vi "ep_Rapid Voltage Changes (1ch).vi"(0 "RMS (1/2) (half cycle)":cluster{"times":timestamp[], "RMS (1/2)":dbl[]}, 1 "init":bool, 5 "RVC settings":T3={"min rate of change [%/sec]"=0.5, "steadiness of steady state [%]"=0.2, "min steady state duration [sec]"=1.0, "min steady state difference [%]"=0.0, "max voltage change [%]"=3.3}, 7 "voltage flag":bool, 9 "nominal voltage [V]":dbl=230.0, 11 "phase":T1, 12 "nominal frequency":enum16{"50 Hz", "60 Hz"}(ring)) -> (4 "rapid voltage changes":T2(array[cluster]), 6 "d(t)":dbl[](array[numeric]))   [LabVIEW 2011, in "NI_EP_Power Quality.lvlib"]
uses:
  <vilib>/addons/Electrical Power/PQ/NI_EP_Power Quality.lvlib
  <vilib>/addons/Electrical Power/PQ/Common/Controls/ep_Phase.ctl
  <vilib>/Analysis/NI_AALBase.lvlib
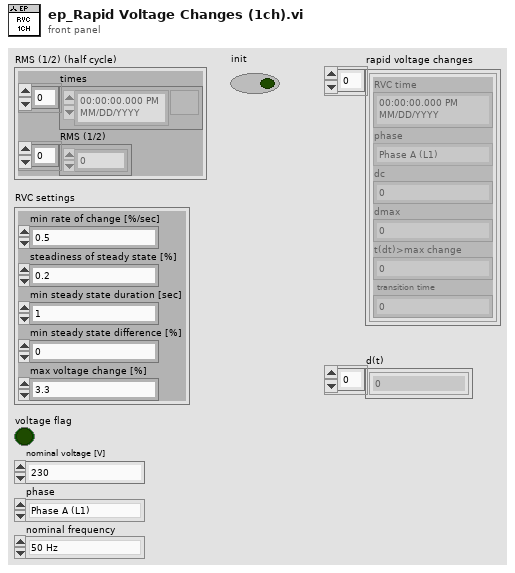
[diagram p1: front panel]
types:
  T1 = typedef "NI_EP_Power Quality.lvlib/ep_Phase.ctl" = enum16{"Phase A (L1)", "Phase B (L2)", "Phase C (L3)", "Phase N", "~3 Phases"}
  T2 = cluster{"RVC time":timestamp, "phase":T1, "dc":dbl, "dmax":dbl, "t(dt)>max change":dbl, " transition time":dbl}[]
  T3 = cluster{"min rate of change [%/sec]":dbl, "steadiness of steady state [%]":dbl, "min steady state duration [sec]":dbl, "min steady state difference [%]":dbl, "max voltage change [%]":dbl}
  T4 = cluster{"event time":timestamp, "phase":T1, "dmax":dbl, "dc":dbl, "duration":dbl, "t(d(t))>":dbl}[]
  T5 = cluster{timestamp, "phase":T1, dbl, dbl, dbl, dbl}
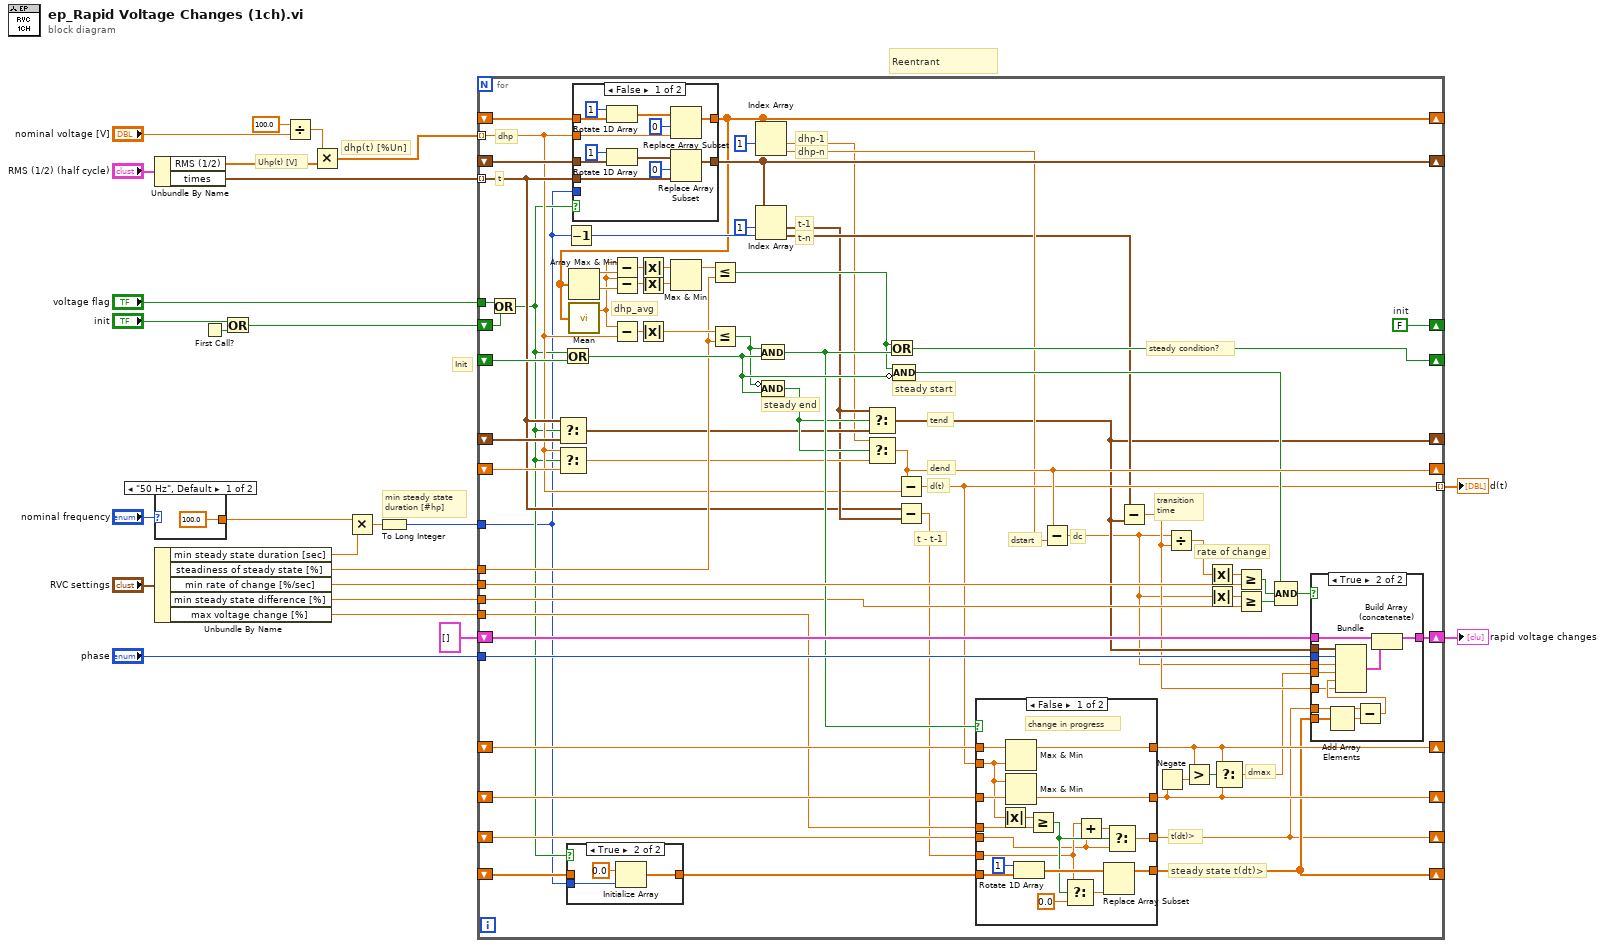
[diagram p0: block diagram]
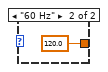
[diagram p2: hidden frame]
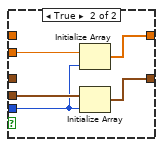
[diagram p4: hidden frame]
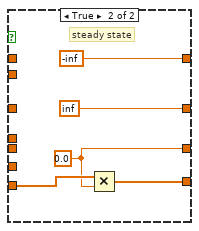
[diagram p6: hidden frame]
diagram:
  # "Init"
  # "min steady state\nduration [#hp]"
  # "dhp(t) [%Un]"
  # "Uhp(t) [V]"
  # "Reentrant"
  n1 = Unbundle By Name("RMS (1/2) (half cycle)") -> ("RMS (1/2)"=w17:dbl[], "times"=w23:timestamp[])
  n2 = case shown="\"50 Hz\", Default" "nominal frequency" {
    tunnel: [100.0 ("x") 120.0 ("x")] -> w11
    frame "50 Hz", Default {
    }
    frame "60 Hz" {
    }
  }
  n3 = Unbundle By Name("RVC settings") -> ("min steady state duration [sec]"=w25:dbl, "steadiness of steady state [%]"=w19:dbl, "min rate of change [%/sec]"=w10:dbl, "min steady state difference [%]"=w20:dbl, "max voltage change [%]"=w21:dbl)
  n4 = First Call?() -> (First Call?: T/F=w3:bool)
  n5 = Or(x="init", y=w3) -> (x .or. y?=w5:bool)
  n6 = Divide(x=100.0, y="nominal voltage [V]") -> (x/y=w15:dbl)
  n7 = Multiply(x=w15, y=w17) -> (x*y=w18:dbl[])
  n8 = Multiply(x=w11, y=w25) -> (x*y=w7:dbl)
  n9 = To Long Integer(number=w7) -> (32bit integer=w24:i32)
  n10 = for {
    shift-right: [w98] -> _
    shift-left: w5 -> [w71]
    tunnel: w19 -> [w68]
    shift-right: [w84] -> _
    shift-left: _ -> [w92]
    shift-right: [w91] -> w12
    shift-left: T4 [] ("rapid voltage changes 2") -> [w90]
    tunnel: "phase" -> [w88]
    shift-right: [w77] -> _
    shift-left: _ -> [w86]
    shift-right: [w78] -> _
    shift-left: _ -> [w87]
    shift-right: [w37] -> _
    shift-left: _ -> [w83]
    tunnel: w20 -> [w60]
    tunnel: w10 -> [w82]
    shift-right: [w38] -> _
    shift-left: _ -> [w75]
    tunnel: "voltage flag" -> [w72]
    tunnel: w18 -> [w41] mode=indexing
    shift-right: [w63] -> _
    shift-left: _ -> [w65]
    tunnel: w21 -> [w61]
    tunnel: [w59] -> w22 mode=indexing
    tunnel: w23 -> [w43] mode=indexing
    shift-right: [w45] -> _
    shift-left: _ -> [w57]
    shift-right: [w33] -> _
    shift-left: _ -> [w55]
    tunnel: w24 -> [w28]
    shift-right: [w50] -> _
    shift-left: _ -> [w54]
    w98 = FALSE  # init
    # "t - t-1"
    # "rate of change"
    # "transition\ntime"
    # "dhp-n"
    # "dhp-1"
    # "t-n"
    # "tend"
    # "t-1"
    # "t"
    # "t(dt)>"
    # "steady state t(dt)>"
    # "dmax"
    # "dc"
    # "dstart"
    # "dhp"
    # "d(t)"
    # "dend"
    # "steady end"
    # "steady start"
    # "steady condition?"
    # "dhp_avg"
    n11 = Or(x=w72, y=w71) -> (x .or. y?=w29:bool)
    n12 = Select(t=w43, s=w29, f=w57) -> (s? t:f=w56:timestamp)
    n13 = Select(t=w41, s=w29, f=w65) -> (s? t:f=w64:dbl)
    n14 = Or(x=w29, y=w92) -> (x .or. y?=w85:bool)
    n15 = Decrement(x=w28) -> (x-1=w52:i32)
    n16 = case shown="True" w29 {
      tunnel: [w99 w101] -> w76
      tunnel: w75 -> [w99 _]
      tunnel: w28 -> [_ w100]
      frame False {
      }
      frame True {
        n17 = Initialize Array(0.0, w100) -> (w101:dbl[])
      }
    }
    n18 = case shown="False" w29 {
      tunnel: w28 -> [_ w116]
      tunnel: w41 -> [w110 w119]
      tunnel: [w109 w118] -> w33
      tunnel: w55 -> [w114 _]
      tunnel: w43 -> [w103 w117]
      tunnel: [w104 w115] -> w50
      tunnel: w54 -> [w105 _]
      frame False {
        n19 = Rotate 1D Array(1:w114, 2:1 ("n")) -> (0:w112:dbl[])
        n20 = Rotate 1D Array(1:w105, 2:1 ("n")) -> (0:w107:timestamp[])
        n21 = Replace Array Subset(array=w112, new element=w110, index=0) -> (w109:dbl[])
        n22 = Replace Array Subset(array=w107, new element=w103, index=0) -> (w104:timestamp[])
      }
      frame True {
        n23 = Initialize Array(w119, w116) -> (w118:dbl[])
        n24 = Initialize Array(w117, w116) -> (w115:timestamp[])
      }
    }
    n25 = Array Max & Min(array=w33) -> (max value=w47:dbl, min value=w46:dbl)  [unwired: 2 out]
    n26 = call <vilib>:"Mean.vi"("X"=w33) -> ("mean"=w32:dbl)  [unwired: 1 out]
    n27 = Subtract(x=w32, y=w47) -> (x-y=w97:dbl)
    n28 = Subtract(x=w32, y=w46) -> (x-y=w96:dbl)
    n29 = Subtract(x=w32, y=w41) -> (x-y=w69:dbl)
    n30 = Absolute Value(x=w97) -> (abs(x)=w94:dbl)
    n31 = Absolute Value(x=w96) -> (abs(x)=w95:dbl)
    n32 = Absolute Value(x=w69) -> (abs(x)=w70:dbl)
    n33 = Max & Min(x=w94, y=w95) -> (max(x,y)=w93:dbl)  [unwired: 1 out]
    n34 = Less Or Equal?(x=w93, y=w68) -> (x <= y?=w66:bool)
    n35 = Less Or Equal?(x=w70, y=w68) -> (x <= y?=w67:bool)
    n36 = Index Array(array=w33, index #1=1 ("index")) -> (element #1=w40:dbl, element #2=w49:dbl)  [unwired: 1 in]
    n37 = Index Array(array=w50, index #1=1 ("index"), index #2=w52) -> (element #1=w44:timestamp, element #2=w48:timestamp)
    n38 = And(x=w67, y=w85) -> (x .and. y?=w73:bool)
    n39 = Compound Arithmetic op=AND(invert w67, w85) -> (w58:bool)
    n40 = Select(t=w44, s=w58, f=w56) -> (s? t:f=w45:timestamp)
    n41 = Select(t=w40, s=w58, f=w64) -> (s? t:f=w63:dbl)
    n42 = Or(x=w66, y=w73) -> (x .or. y?=w84:bool)
    n43 = Compound Arithmetic op=AND(w66, invert w85) -> (w62:bool)
    n44 = Subtract(x=w63, y=w41) -> (x-y=w59:dbl)
    n45 = Subtract(x=w43, y=w44) -> (x-y=w42:dbl)
    n46 = case shown="False" w73 {
      tunnel: [w149 -inf] -> w77
      tunnel: w86 -> [w150 _]
      tunnel: w59 -> [w145 _]
      tunnel: [w148 inf] -> w78
      tunnel: w87 -> [w147 _]
      tunnel: w61 -> [w146 _]
      tunnel: [w144 w151] -> w37
      tunnel: w83 -> [w133 _]
      tunnel: w76 -> [w142 w153]
      tunnel: [w139 w152] -> w38
      tunnel: w42 -> [w134 _]
      frame False {
        # "change in progress"
        n47 = Absolute Value(x=w145) -> (abs(x)=w143:dbl)
        n48 = Max & Min(x=w150, y=w145) -> (max(x,y)=w149:dbl)  [unwired: 1 out]
        n49 = Max & Min(x=w145, y=w147) -> (min(x,y)=w148:dbl)  [unwired: 1 out]
        n50 = Rotate 1D Array(1:w142, 2:1 ("n")) -> (0:w140:dbl[])
        n51 = Greater Or Equal?(x=w143, y=w146) -> (x >= y?=w137:bool)
        n52 = Select(t=w134, s=w137, f=0.0) -> (s? t:f=w135:dbl)
        n53 = Add(x=w134, y=w133) -> (x+y=w138:dbl)
        n54 = Replace Array Subset(array=w140, new element=w135) -> (w139:dbl[])  [unwired: 1 in]
        n55 = Select(t=w138, s=w137, f=w133) -> (s? t:f=w144:dbl)
      }
      frame True {
        w151 = 0.0
        # "steady state"
        n56 = Multiply(x=w153, y=w151) -> (x*y=w152:dbl[])
      }
    }
    n57 = Subtract(x=w63, y=w49) -> (x-y=w31:dbl)
    n58 = Subtract(x=w48, y=w45) -> (x-y=w39:dbl)
    n59 = Negate(x=w78) -> (-x=w80:dbl)
    n60 = Divide(x=w31, y=w39) -> (x/y=w30:dbl)
    n61 = Greater?(x=w77, y=w80) -> (0:w79:bool)
    n62 = Absolute Value(x=w30) -> (abs(x)=w34:dbl)
    n63 = Absolute Value(x=w31) -> (abs(x)=w35:dbl)
    n64 = Select(t=w77, s=w79, f=w78) -> (s? t:f=w36:dbl)
    n65 = Greater Or Equal?(x=w34, y=w82) -> (x >= y?=w81:bool)
    n66 = Greater Or Equal?(x=w35, y=w60) -> (x >= y?=w74:bool)
    n67 = Compound Arithmetic op=AND(w62, w81, w74) -> (w89:bool)
    n68 = case shown="True" w89 {
      tunnel: w45 -> [_ w126]
      tunnel: w88 -> [_ w132]
      tunnel: w31 -> [_ w131]
      tunnel: w36 -> [_ w130]
      tunnel: w39 -> [_ w121]
      tunnel: w90 -> [w120 w128]
      tunnel: [w120 w127] -> w91
      tunnel: w37 -> [_ w124]
      tunnel: w38 -> [_ w123]
      frame False {
      }
      frame True {
        n69 = Add Array Elements(numeric array=w123) -> (sum=w125:dbl)
        n70 = Subtract(x=w124, y=w125) -> (x-y=w122:dbl)
        n71 = Bundle(w126, "phase"=w132, w131, w130, w122, w121) -> (w129:T5)  [unwired: 1 in]
        n72 = Build Array (concatenate)(w128, w129) -> (w127:T4)
      }
    }
  }
  "rapid voltage changes" <- w12
  "d(t)" <- w22
